vi "仪器面板_计数判断处理.vi"(1 "数值":dbl) -> (0 "数值 2":dbl)   [LabVIEW 2014]
panel:
  out "x":dbl
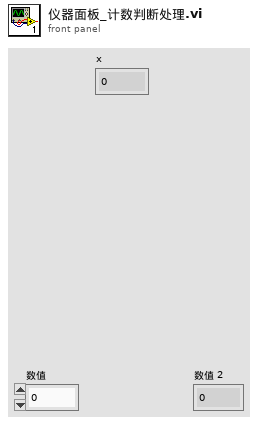
[diagram p1: front panel]
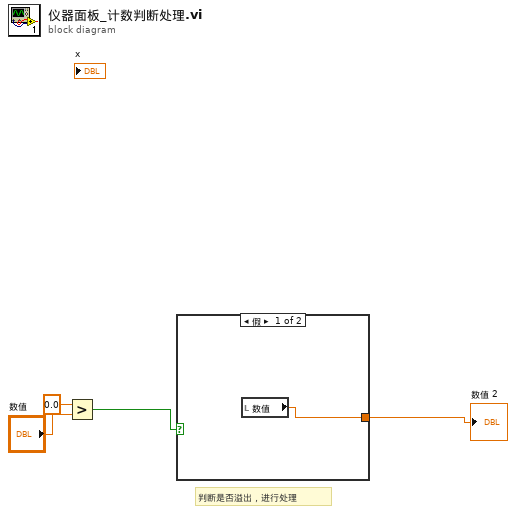
[diagram p0: block diagram]
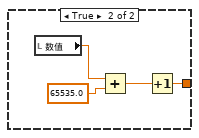
[diagram p2: hidden frame]
diagram:
  # "判断是否溢出，进行处理"
  n1 = Greater?(x=0.0, y="数值") -> (0:w2:bool)
  n2 = case shown="假" w2 {
    tunnel: [w5 w6] -> w1
    frame False {
      n3 = local read "数值"() -> (w5:dbl)
    }
    frame True {
      n4 = local read "数值"() -> (w7:dbl)
      n5 = Add(x=w7, y=65535.0) -> (x+y=w9:dbl)
      n6 = Increment(x=w9) -> (x+1=w6:dbl)
    }
  }
  "数值 2" <- w1
